vi "sub_resample_and_demodulate.vi"() -> ()   [LabVIEW 2019]
uses:
  <vilib>/addons/Modulation/Analog/controls/Complex Data Waveform.ctl
  <vilib>/addons/Modulation/niAMT.lvlib
  <vilib>/addons/Modulation/niDMT.lvlib
panel:
  out "Waveform":dbl[][](graph)
  out "Waveform 2":dbl[][](graph)
  out "Waveform 3":dbl[][](graph)
  out "Sync Found":bool
  out "output bit stream":i8[][](array[numeric])
  in  "Rx IQ Sampling\nRate [s/sec]":dbl
  in  "packet_arr":cdb[][](array[numeric])
  in  "PSK Init Parameters":T1
  out "recovered complex waveform":T2[](array[typedef]) {"Y" format="%.3f"; "dt" format="%^.2e"; "t0" format="%.4f"}
  in  "error in (no error)":errorcluster
  out "error out":errorcluster
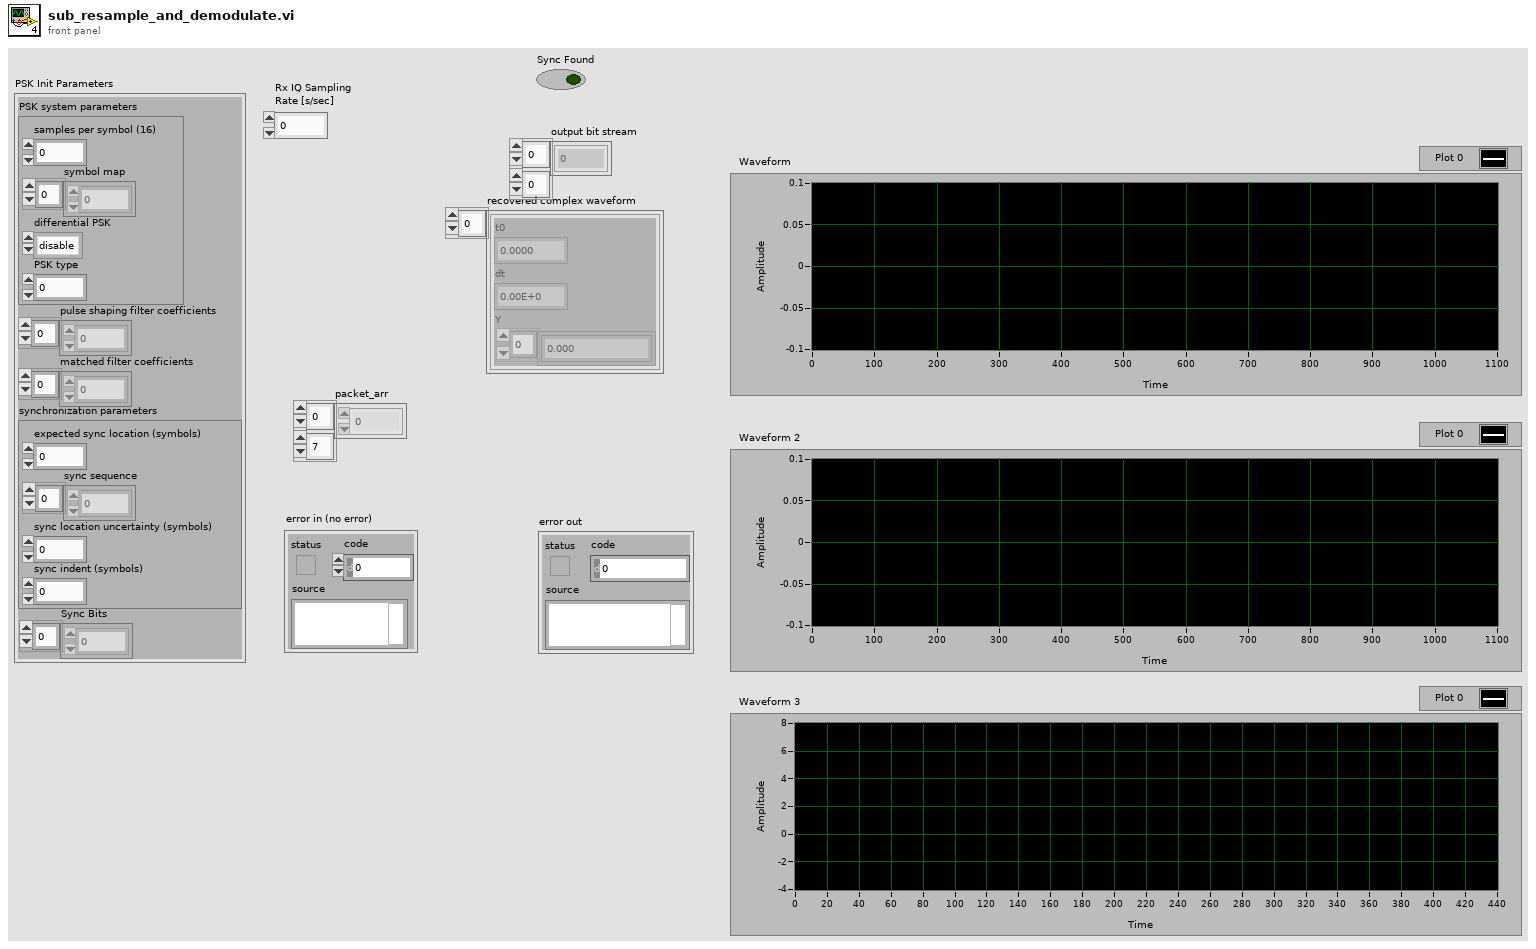
[diagram p1: front panel]
types:
  T1 = cluster{"PSK system parameters":cluster{"samples per symbol (16)":i32, "symbol map":cdb[], "differential PSK":enum16{"disable", "enable"}, "PSK type":u16}, "pulse shaping filter coefficients":dbl[], "matched filter coefficients":dbl[], "synchronization parameters":cluster{"expected sync location (symbols)":i32, "sync sequence":cdb[], "sync location uncertainty (symbols)":i32, "sync indent (symbols)":i32}, "Sync Bits":i8[]}
  T2 = typedef "niAMT.lvlib/Complex Data Waveform.ctl" = cluster{"t0":dbl, "dt":dbl, "Y":cdb[]}
  T3 = cluster{"samples per symbol (16)":i32, "symbol map":cdb[], "differential PSK":enum16{"disable", "enable"}, "PSK type":u16}
  T4 = cluster{"expected sync location (symbols)":i32, "sync sequence":cdb[], "sync location uncertainty (symbols)":i32, "sync indent (symbols)":i32}
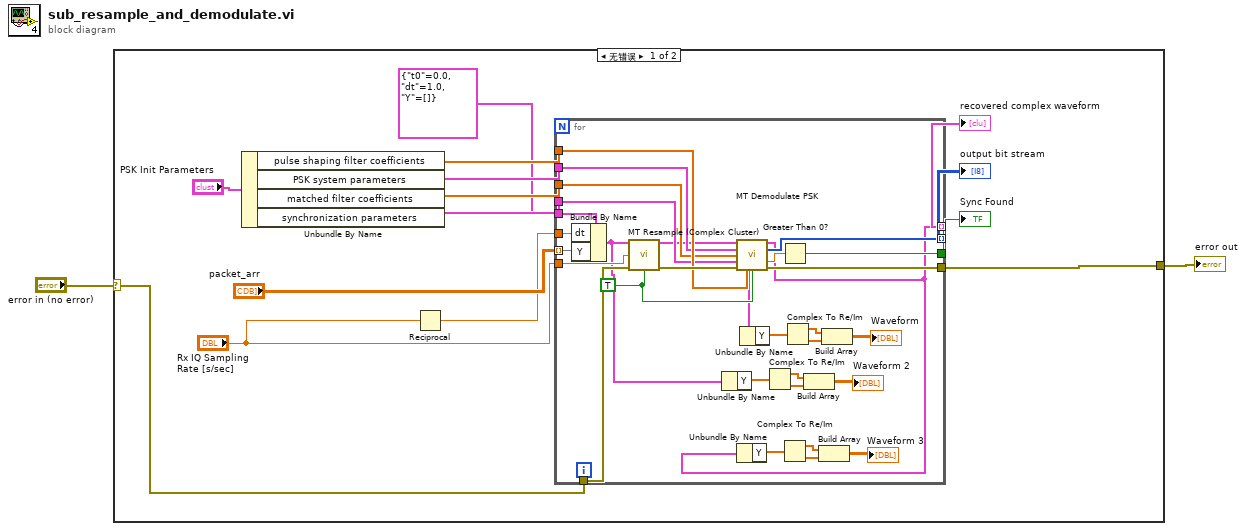
[diagram p0: block diagram]
diagram:
  n1 = case shown="无错误" "error in (no error)" {
    selector: "error in (no error)" -> [w3 w47]
    tunnel: [w13 w47] -> w2
    frame No Error {
      n2 = Unbundle By Name("PSK Init Parameters") -> ("pulse shaping filter coefficients"=w8:dbl[], "PSK system parameters"=w11:T3, "matched filter coefficients"=w10:dbl[], "synchronization parameters"=w9:T4)
      n3 = Reciprocal(x="Rx IQ Sampling\nRate [s/sec]") -> (1/x=w5:dbl)
      n4 = for {
        tunnel: "packet_arr" -> [w32] mode=indexing
        tunnel: "Rx IQ Sampling\nRate [s/sec]" -> [w45]
        tunnel: w8 -> [w44]
        tunnel: w10 -> [w43]
        tunnel: w11 -> [w42]
        tunnel: [w41] -> w15 mode=indexing
        tunnel: w9 -> [w40]
        tunnel: [w38] -> w16
        tunnel: [w37] -> w13
        tunnel: [w17] -> w7 mode=indexing
        tunnel: w5 -> [w35]
        tunnel: T2 {"t0"=0.0, "dt"=1.0, "Y"=[]} ("input complex waveform") -> [w34]
        tunnel: w3 -> [w33]
        w36 = TRUE ("reset? (T)")
        n5 = Bundle By Name(cluster=w34, "dt"=w35, "Y"=w32) -> (w22:T2)
        n6 = call <vilib>:"MT Resample (Complex Cluster).vi"("input complex waveform"=w22, "desired sample rate (Hz)"=w45, "error in (no error)"=w33, "reset? (T)"=w36) -> ("output complex waveform"=w31:T2, "error out"=w46:errorcluster)  [unwired: 10 in]
        n7 = Unbundle By Name(w22) -> ("Y"=w26:cdb[])
        n8 = call <vilib>:"MT Demodulate PSK.vi"("input complex waveform"=w31, "PSK system parameters"=w42, "matched filter coefficients"=w43, "synchronization parameters"=w40, "error in (no error)"=w46, "pulse shaping filter coefficients"=w44, "reset? (T)"=w36) -> ("recovered complex waveform"=w17:T2, "output bit stream"=w41:i8[], "sync found index (symbols)"=w39:dbl, "error out"=w37:errorcluster)  [unwired: 4 in, 1 out]
        n9 = Unbundle By Name(w17) -> ("Y"=w21:cdb[])
        n10 = Unbundle By Name(w31) -> ("Y"=w30:cdb[])
        n11 = Complex To Re/Im(x + iy=w26) -> (x=w24:dbl[], y=w23:dbl[])
        n12 = Greater Than 0?(x=w39) -> (x > 0?=w38:bool)
        n13 = Complex To Re/Im(x + iy=w21) -> (x=w19:dbl[], y=w18:dbl[])
        n14 = Complex To Re/Im(x + iy=w30) -> (x=w28:dbl[], y=w27:dbl[])
        n15 = Build Array(w24, w23) -> (→"Waveform 2":dbl[][])
        n16 = Build Array(w19, w18) -> (→"Waveform 3":dbl[][])
        n17 = Build Array(w28, w27) -> (→"Waveform":dbl[][])
      }
      "Sync Found" <- w16
      "output bit stream" <- w15
      "recovered complex waveform" <- w7
    }
    frame Error {
    }
  }
  "error out" <- w2
